vi "tm483_masterpulse.vi"() -> ()   [LabVIEW 2011]
panel:
  in  "Interval":dbl=0.5
  out "DCAM Version":string
  out "Library Version":string
  out "Image":u16[][](graph)
  out "Frames Per Second":dbl
  in  "Quit":bool
  out "Error Out":errorcluster {"code" format="%.0x"}
  # "This example will demonstrate how to configure the master pulse and use it for internal trigger capture.  The master pulse signal is also sent to the output trigger in this example."
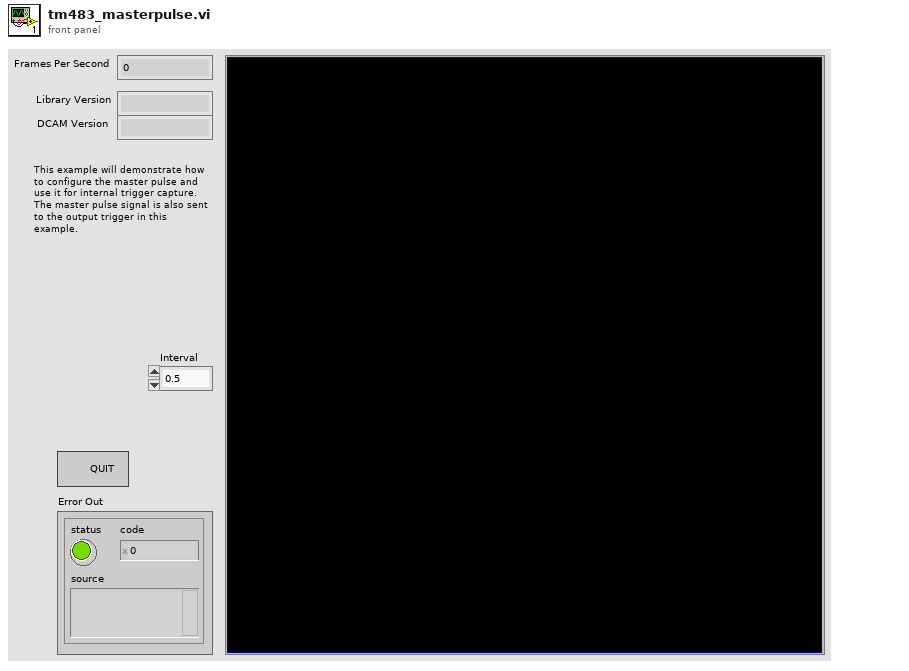
[diagram p1: front panel]
types:
  T1 = cluster{"Capture Library":string, "DCAM-API":string}
  T2 = cluster{"Mode":u32, "Polarity":u32, "Times":u32, "Delay":dbl}
  T3 = cluster{"Mode":u32, "Source":u32, "Interval":dbl, "Burst":u32}
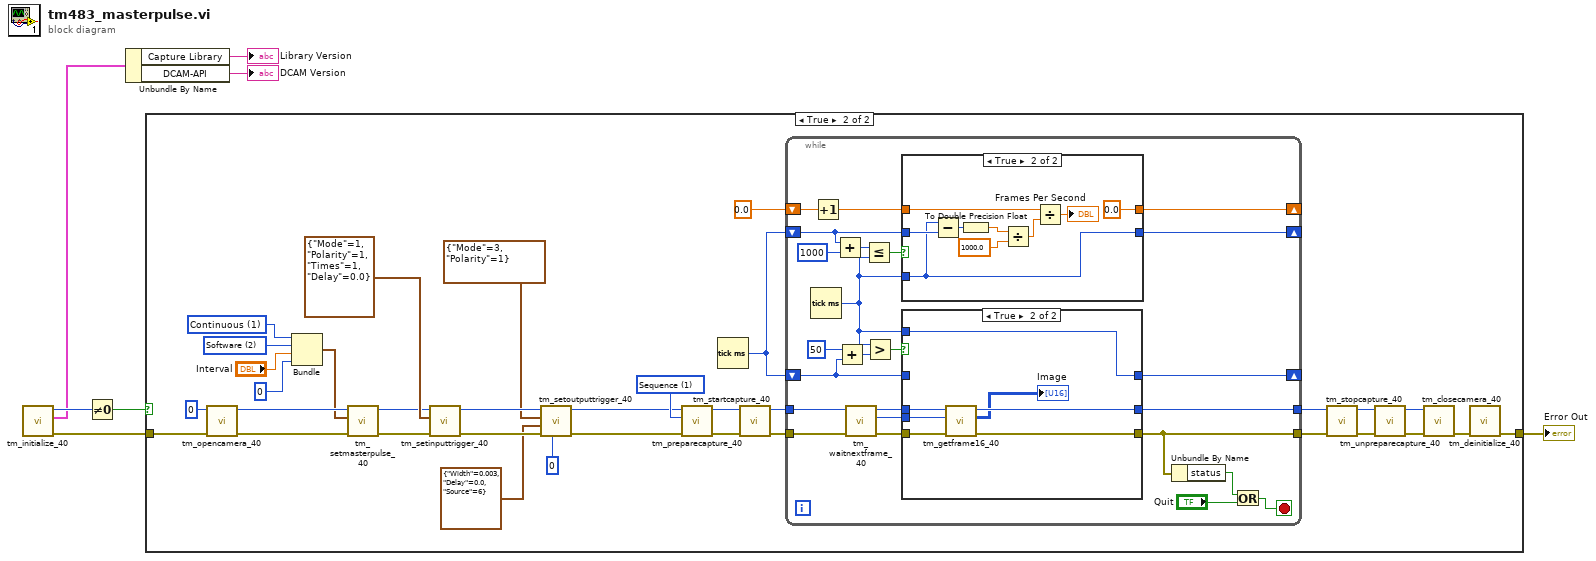
[diagram p0: block diagram]
diagram:
  n1 = call <userlib>:"tm_initialize_40.vi"() -> ("error out"=w4:errorcluster, "Version Info"=w3:T1, "Number Of Cameras"=w5:u32)  [unwired: 8 in, 1 out]
  n2 = Not Equal To 0?(x=w5) -> (x != 0?=w7:bool)
  n3 = Unbundle By Name(w3) -> ("Capture Library"=→"Library Version":string, "DCAM-API"=→"DCAM Version":string)
  n4 = case shown="True" w7 {
    tunnel: w4 -> [w8 w42]
    tunnel: [w8 w39] -> w6
    frame False {
    }
    frame True {
      w22 = u32 2 items=["External"=1, "Software"=2] ("Source")
      w23 = u32 1 items=["Continuous"=1, "Start"=2, "Burst"=3] ("Mode")
      w30 = 1 items=["Snap", "Sequence"] ("Capture mode")
      n5 = call <userlib>:"tm_opencamera_40.vi"("error in (no error)"=w42, "Camera Index"=u32 0) -> ("error out"=w24:errorcluster, "Handle out"=w25:u32)  [unwired: 7 in, 1 out]
      n6 = Bundle("Mode"=w23, "Source"=w22, "Interval"="Interval", "Burst"=u32 0) -> (w20:T3)  [unwired: 1 in]
      n7 = call <userlib>:"tm_setmasterpulse_40.vi"("error in (no error)"=w24, "Parameters"=w20, "Handle in"=w25) -> ("error out"=w17:errorcluster, "Handle out"=w16:u32)  [unwired: 7 in]
      n8 = call <userlib>:"tm_setinputtrigger_40.vi"("error in (no error)"=w17, "Parameters"=T2 {"Mode"=1, "Polarity"=1, "Times"=1, "Delay"=0.0}, "Handle in"=w16) -> ("error out"=w15:errorcluster, "Handle out"=w14:u32)  [unwired: 7 in]
      n9 = call <userlib>:"tm_setoutputtrigger_40.vi"("Port"=0, "error in (no error)"=w15, "Programmable Options"=cluster{"Width":dbl, "Delay":dbl, "Source":u32} {"Width"=0.003, "Delay"=0.0, "Source"=6}, "Type"=cluster{"Mode":u32, "Polarity":u32} {"Mode"=3, "Polarity"=1}, "Handle in"=w14) -> ("error out"=w11:errorcluster, "Handle out"=w10:u32)  [unwired: 5 in]
      n10 = call <userlib>:"tm_preparecapture_40.vi"("error in (no error)"=w11, "Capture mode"=w30, "Handle in"=w10) -> ("error out"=w28:errorcluster, "Handle out"=w29:u32)  [unwired: 5 in, 2 out]
      n11 = Tick Count (ms)() -> (millisecond timer value=w26:u32)
      n12 = call <userlib>:"tm_startcapture_40.vi"("error in (no error)"=w28, "Handle in"=w29) -> ("error out"=w31:errorcluster, "Handle out"=w32:u32)  [unwired: 8 in]
      n13 = while {
        tunnel: [w45] -> w35
        tunnel: [w46] -> w36
        tunnel: w32 -> [w63]
        tunnel: w31 -> [w64]
        shift-right: [w61] -> _
        shift-left: w26 -> [w58]
        shift-right: [w62] -> _
        shift-left: 0.0 -> [w55]
        shift-right: [w44] -> _
        shift-left: w26 -> [w47]
        stop <- w43 stop-if-true
        n14 = Tick Count (ms)() -> (millisecond timer value=w48:u32)
        n15 = Increment(x=w55) -> (x+1=w56:dbl)
        n16 = Add(x=w58, y=u32 1000) -> (x+y=w60:u32)
        n17 = Add(x=u32 50, y=w47) -> (x+y=w50:u32)
        n18 = call <userlib>:"tm_waitnextframe_40.vi"("error in (no error)"=w64, "Handle in"=w63) -> ("error out"=w53:errorcluster, "Frame Index"=w52:i32, "Handle out"=w54:u32)  [unwired: 6 in, 1 out]
        n19 = Less Or Equal?(x=w60, y=w48) -> (x <= y?=w57:bool)
        n20 = Greater?(x=w48, y=w50) -> (0:w49:bool)
        n21 = case shown="True" w57 {
          tunnel: w58 -> [w78 w81]
          tunnel: [w78 w79] -> w61
          tunnel: w56 -> [w77 w85]
          tunnel: w48 -> [_ w79]
          tunnel: [w77 0.0] -> w62
          frame False {
          }
          frame True {
            n22 = Subtract(x=w79, y=w81) -> (x-y=w80:u32)
            n23 = To Double Precision Float(number=w80) -> (double precision float=w87:dbl)
            n24 = Divide(x=w87, y=1000.0) -> (x/y=w84:dbl)
            n25 = Divide(x=w85, y=w84) -> (x/y=→"Frames Per Second":dbl)
          }
        }
        n26 = case shown="True" w49 {
          tunnel: w54 -> [w69 w76]
          tunnel: w53 -> [w68 w75]
          tunnel: w52 -> [_ w74]
          tunnel: w47 -> [w67 _]
          tunnel: w48 -> [_ w73]
          tunnel: [w69 w71] -> w45
          tunnel: [w68 w72] -> w46
          tunnel: [w67 w73] -> w44
          frame False {
          }
          frame True {
            n27 = call <userlib>:"tm_getframe16_40.vi"("error in (no error)"=w75, "Frame Index"=w74, "Handle in"=w76) -> ("error out"=w72:errorcluster, "Data"=→"Image":u16[][], "Handle out"=w71:u32)  [unwired: 5 in, 1 out]
          }
        }
        n28 = Unbundle By Name(w46) -> ("status"=w66:bool)
        n29 = Or(x=w66, y="Quit") -> (x .or. y?=w43:bool)
      }
      n30 = call <userlib>:"tm_stopcapture_40.vi"("error in (no error)"=w36, "Handle in"=w35) -> ("error out"=w33:errorcluster, "Handle out"=w34:u32)  [unwired: 8 in]
      n31 = call <userlib>:"tm_unpreparecapture_40.vi"("error in (no error)"=w33, "Handle in"=w34) -> ("error out"=w38:errorcluster, "Handle out"=w37:u32)  [unwired: 8 in]
      n32 = call <userlib>:"tm_closecamera_40.vi"("error in (no error)"=w38, "Handle in"=w37) -> ("error out"=w40:errorcluster)  [unwired: 9 in]
      n33 = call <userlib>:"tm_deinitialize_40.vi"("error in (no error)"=w40) -> ("error out"=w39:errorcluster)  [unwired: 10 in]
    }
  }
  "Error Out" <- w6
